vi "Teardown.vi"(11 "Dev Panel in":refnum<class "Dev Panel.lvclass">) -> (3 "Dev Panel out":refnum<class "Dev Panel.lvclass">)   [LabVIEW 2021, in "Dev Panel.lvclass"]
uses:
  Dev Panel.lvclass
  Dev Panel.lvclass/Dev Panel.ctl
  Actor/Event Actor/Event Actor.lvclass
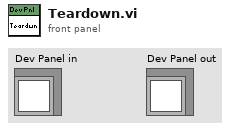
[diagram p1: front panel]
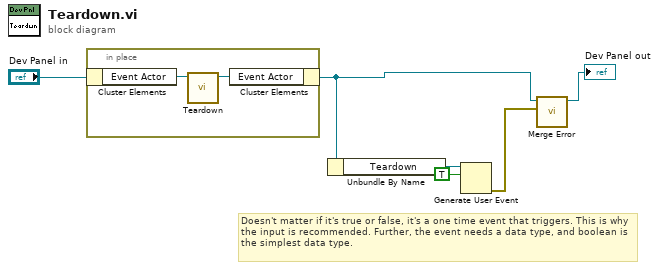
[diagram p0: block diagram]
diagram:
  # "Doesn't matter if it's true or false, it's a one time event that triggers. This is why the input is recommended. Further, the event needs a data type, and boolean is the simplest data type."
  n1 = in-place {
    n2 = in-place-cluster #1("Dev Panel in") -> ("Event Actor"=w8:refnum<class "Event Actor.lvclass">)
    n3 = call-dynamic "Teardown.vi"("Teardown in"=w8) -> ("Teardown out"=w7:refnum<class "Event Actor.lvclass">)  [unwired: 10 in]
    n4 = in-place-cluster #1("Event Actor"=w7) -> (w3:refnum<class "Dev Panel.lvclass">)
  }
  n5 = Unbundle By Name(w3) -> ("Teardown"=w4:refnum<user-event>)
  n6 = Generate User Event(user event=w4, event data cluster=TRUE ("event data")) -> (error out=w1:errorcluster)  [unwired: 2 in, 1 out]
  n7 = call-dynamic "Merge Error.vi"("Error"=w1, "Set Error in"=w3) -> ("Set Error out"=→"Dev Panel out":refnum<class "Dev Panel.lvclass">)  [unwired: 9 in]
